vi "Initial Matrix (CDB).vi"(10 "column":i32, 11 "row":i32) -> (0 "error":i32, 3 "Matrix":T1)   [LabVIEW 2014, in "NI_AALBase.lvlib"]
uses:
  NI_AALBase.lvlib
  ComplexMatrix.ctl
  lvanlys.dll
  NI_Matrix.lvlib
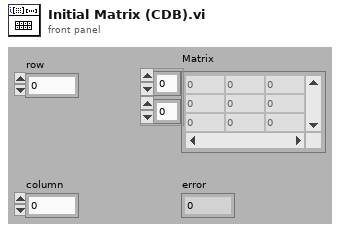
[diagram p1: front panel]
types:
  T1 = typedef "NI_Matrix.lvlib/ComplexMatrix.ctl" = cdb[][]
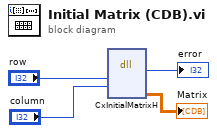
[diagram p0: block diagram]
diagram:
  n1 = dll-call lib="C:/Program Files (x86)/National Instruments/LabVIEW 2014/resource/lvanlys.*" fn="CxInitialMatrixH"("row"="row", "col"="column") -> (→"error":i32, "Matrix"=→"Matrix":T1)  [unwired: 6 in, 2 out]
